vi "Timing.Set Offset.vi"(10 "Offset":u64, 11 "Timing in":refnum<class "Timing.lvclass">) -> (3 "Timing out":refnum<class "Timing.lvclass">)   [LabVIEW 2017, in "DSF Core.lvlib" / "Timing.lvclass"]
uses:
  Timing.lvclass
  Timing.lvclass/Timing.ctl
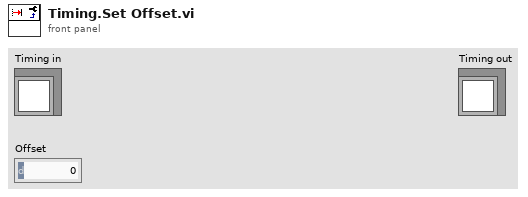
[diagram p1: front panel]
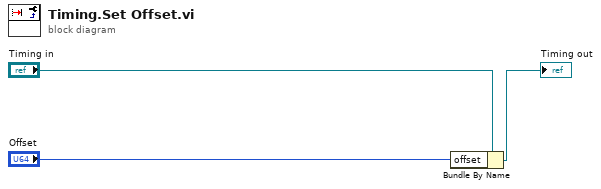
[diagram p0: block diagram]
diagram:
  n1 = Bundle By Name(cluster="Timing in", "offset"="Offset") -> (→"Timing out":refnum<class "Timing.lvclass">)
